vi "Quick Usb Read Data Async.vi"(0 "hDevice":u32, 5 "data":string, 7 "length":u32, 9 "transaction":string, 11 "error in (no error)":errorcluster) -> (3 "function return":i32, 4 "hDevice out":u32, 6 "data out":string, 8 "length out":u32, 10 "transaction out":string, 15 "error out":errorcluster)   [LabVIEW 2011, in "QuickUSB.lvlib"]
doc: "QUSBLIB QRETURN QuickUsbReadDataAsync(\n QHANDLE hDevice, \n PQBYTE data, \n PQULONG length, \n PQBYTE transaction\n);"
uses:
  QuickUSB.lvlib
  QuickUSB.dll
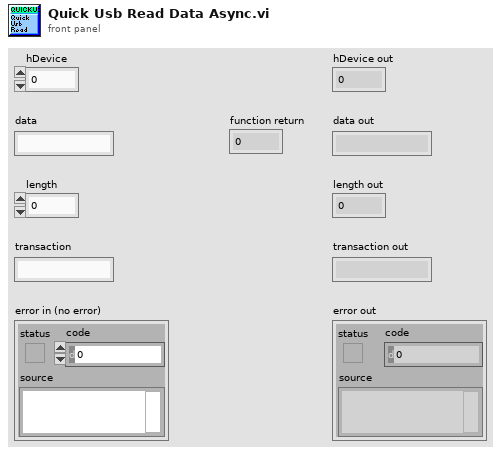
[diagram p1: front panel]
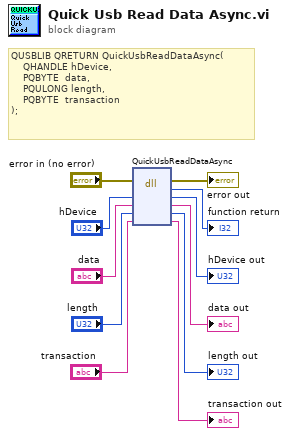
[diagram p0: block diagram]
diagram:
  # "QUSBLIB QRETURN QuickUsbReadDataAsync(\n    QHANDLE hDevice, \n    PQBYTE  data, \n    PQULONG length, \n    PQBYTE  transaction\n);"
  n1 = dll-call lib="C:/QuickUSB/QuickUSB.*" fn="QuickUsbReadDataAsync"(error in="error in (no error)", "hDevice"="hDevice", "data"="data", "length"="length", "transaction"="transaction") -> (error out=→"error out":errorcluster, →"function return":i32, "hDevice"=→"hDevice out":u32, "data"=→"data out":string, "length"=→"length out":u32, "transaction"=→"transaction out":string)  [unwired: 2 in, 1 out]
